vi "Linear.vi"(0 "VISA resource name":refnum<visa-resource-name>, 7 "Channel (1)":i32=1 min=1 max=16 step=1, 11 "error in (no error)":errorcluster) -> (4 "VISA resource name out":refnum<visa-resource-name>, 8 "Linear Value":dbl min=-100000000.0 max=100000000.0 step=1e-05 format="%^.5e", 15 "error out":errorcluster)   [LabVIEW 2012, in "Lake Shore Cryotronics 370.lvlib"]
doc: "This VI querys the instrument for linear equation data for the selected channel."
uses:
  <instrlib>/Lake Shore Cryotronics 370/Lake Shore Cryotronics 370.lvlib
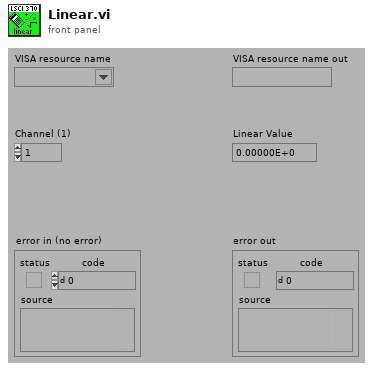
[diagram p1: front panel]
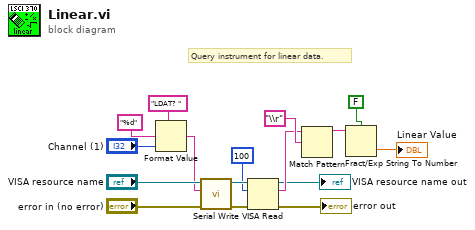
[diagram p0: block diagram]
diagram:
  # "Query instrument for linear data."
  n1 = Format Value(string ("")="LDAT? ", format string="%d", value (0)="Channel (1)") -> (output string=w1:string)
  n2 = call <instrlib>:"Serial Write.vi"("error in (no error)"="error in (no error)", "Write Buffer (\"\")"=w1, "VISA resource name"="VISA resource name") -> ("error out"=w15:errorcluster, "VISA resource name out"=w16:refnum<visa-resource-name>)  [unwired: 6 in, 1 out]
  n3 = VISA Read(VISA resource name=w16, byte count=100, error in (no error)=w15) -> (VISA resource name out=→"VISA resource name out":refnum<visa-resource-name>, read buffer=w13:string, error out=→"error out":errorcluster)  [unwired: 1 out]
  n4 = Match Pattern(string=w13, regular expression="\\r") -> (before substring=w11:string)  [unwired: 1 in, 3 out]
  n5 = Fract/Exp String To Number(use system decimal point (T)=FALSE, string=w11) -> (number=→"Linear Value":dbl)  [unwired: 2 in, 1 out]
